vi "PathPlanner_Read_Path_FIle_Global_Example.vi"() -> ()   [LabVIEW 2019]
uses:
  SubVI/pathplanner_read_path_GlobalVariable.vi
  <vilib>/Rock Robotics/WPI/ThirdParty/JAS_Junk/TrajLib/TypeDef/CHASSIS_SPEEDS.ctl
  <vilib>/Rock Robotics/WPI/ThirdParty/JAS_Junk/TrajLib/Trajectory_Library.lvlib
panel:
  in  "StartingSpeeds":T1 {"vOmega" format="%10.3f"; "vY" format="%10.3f"; "vX" format="%10.3f"}
  out "error out":errorcluster
  # "Read PATH File and \nWrite to Global Variable"
  # "See block diagram"
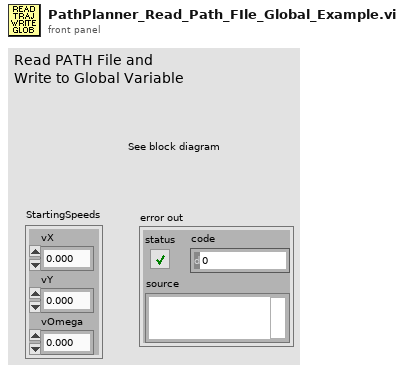
[diagram p1: front panel]
types:
  T1 = typedef "Trajectory_Library.lvlib/CHASSIS_SPEEDS.ctl" = cluster{"vX":dbl, "vY":dbl, "vOmega":dbl}
  T2 = typedef "PathPlanner24.lvlib/PathPlannerTrajectory.ctl" = cluster{"States":T3[]}
  T3 = typedef "PathPlanner24.lvlib/PathPlannerTrajectoryState.ctl" = cluster{"TimeSeconds":dbl, "VelocityMPS":dbl, "AccerationMpsSq":dbl, "HeadingAngularVelRadPerSec":dbl, "PositionMeters":T4, "Heading":T5, "TargetHolonomicRotation":T5, "CurvatureRadPerMeter":dbl, "PathPlannerConstraints":T6, "DeltaPos":dbl}
  T4 = typedef "Trajectory_Library.lvlib/TRANSLATION2D.ctl" = cluster{"X":dbl, "Y":dbl}
  T5 = typedef "Trajectory_Library.lvlib/ROTATION2D.ctl" = cluster{"VALUE":dbl, "COS":dbl, "SIN":dbl}
  T6 = typedef "PathPlanner24.lvlib/PathPlannerPathConstraints.ctl" = cluster{"MaxVelocityMps;":dbl, "MaxAccelerationMpsSq;":dbl, "MaxAngularVelRadPsEc;":dbl, "MaxAngularAccRadPSecSq":dbl, "Exists":bool}
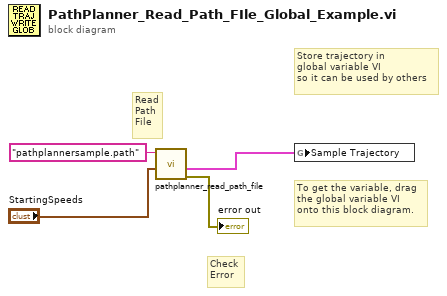
[diagram p0: block diagram]
diagram:
  # "Check\nError"
  # "Read\nPath\nFile"
  # "To get the variable, drag\nthe global variable VI\nonto this block diagram."
  # "Store trajectory in\nglobal variable VI\nso it can be used by others"
  n1 = call "pathplanner_read_path_file.vi"("StartingSpeeds"="StartingSpeeds", "Path File Name"="pathplannersample.path" ("CSV File Name")) -> ("error out"=→"error out":errorcluster, "Path Planner Trajectory"=w2:T2)  [unwired: 6 in, 2 out]
  n2 = global write "pathplanner_read_path_GlobalVariable.vi" "Sample Trajectory"(w2) -> ()
